vi "PPG_ABC.start ABC.vi"(0 "i ref in":refnum<vi>, 2 "patternGroup":i32, 3 "ms timeout [ms]":i32=10000, 5 "error in (no error)":errorcluster) -> (14 "i ref out":refnum<vi>, 17 "timed out":bool, 19 "error out":errorcluster)   [LabVIEW 2014, in "PPG_ABC.lvlib"]
doc: "Starts execution for the specified pattern group."
uses:
  PPG_ABC.lvlib
  PPG_ABC.PG_Running.ctl
  NI_FPGA_PPG/NI_FPGA_PPG.lvlib
  CSlibraries/UtilityLib/UtilityLib.lvlib
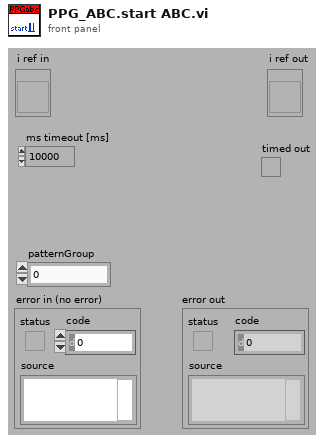
[diagram p1: front panel]
types:
  T1 = typedef "PPG_ABC.lvlib/PPG_ABC.PG_Running.ctl" = i32
  T2 = typedef "PPG_ABC.lvlib/PPG_ABC.i attribute.ctl" = cluster{"patternGroups":T3[], "defaultLetter":string, "defaultPatternGroup":i32, "PGRunning":T1, "PGRunningID":i32, "pgStarting":T4}
  T3 = typedef "PPG_ABC.lvlib/PPG_ABC.PG_dataType.ctl" = cluster{"PGDevice":string, "rawPatternData":cluster{"triggerCondition":i32, "timeTable":dbl[], "channelTable":string[]}[]}
  T4 = typedef "Semaphore RefNum" = refnum<k1>
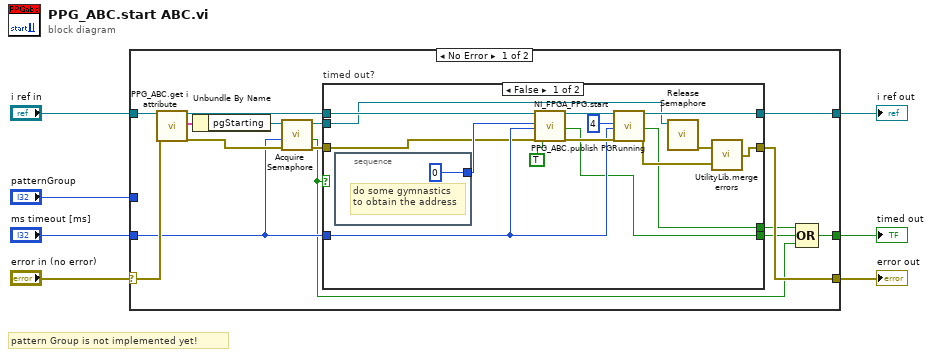
[diagram p0: block diagram]
diagram:
  # "pattern Group is not implemented yet!"
  n1 = case shown="No Error" "error in (no error)" {
    selector: "error in (no error)" -> [w19 w42]
    tunnel: [w21 w42] -> w6
    tunnel: "i ref in" -> [w20 w41]
    tunnel: [w22 w41] -> w4
    tunnel: [w10 _] -> w3
    tunnel: "ms timeout [ms]" -> [w12 _]
    tunnel: "patternGroup" -> [_ _]
    frame No Error {
      n2 = call "PPG_ABC.get i attribute.vi"("i ref in"=w20, "error in (no error)"=w19) -> ("i ref out"=w15:refnum<vi>, "i attribute"=w18:T2, "error out"=w16:errorcluster)  [unwired: 15 in]
      n3 = Unbundle By Name(w18) -> ("pgStarting"=w17:T4)
      n4 = call <vilib>:"Acquire Semaphore.vi"("error in (no error)"=w16, "ms timeout (-1)"=w12, "semaphore"=w17) -> ("error out"=w14:errorcluster, "timed out"=w11:bool, "semaphore out"=w13:T4)  [unwired: 2 in]
      n5 = case "timed out?" shown="False" w11 {
        tunnel: [w35 w40] -> w22
        tunnel: [w26 w39] -> w21
        tunnel: w12 -> [w33 _]
        tunnel: w15 -> [w31 w40]
        tunnel: w14 -> [w29 w39]
        tunnel: w13 -> [w30 _]
        tunnel: [w25 _] -> w9
        tunnel: [w24 _] -> w8
        frame False {
          n6 = stacked-sequence {
            tunnel: [0 ("start_addr")] -> w37
            frame #0 {
              # "do some gymnastics\nto obtain the address"
            }
          }
          n7 = call "NI_FPGA_PPG.start.vi"("i ref in"=w31, "start_addr"=w37, "ms timeout (10000)"=w33, "error in (no error)"=w29, "ignorePdcHandling"=TRUE) -> ("i ref out"=w36:refnum<vi>, "timed out"=w24:bool, "error out"=w34:errorcluster)  [unwired: 12 in]
          n8 = call "PPG_ABC.publish PGRunning.vi"("i ref in"=w36, "PPGRunning"=T1 4, "ms timeout (10000)"=w33, "error in (no error)"=w34) -> ("i ref out"=w35:refnum<vi>, "timed out"=w25:bool, "error out"=w27:errorcluster)  [unwired: 13 in]
          n9 = call <vilib>:"Release Semaphore.vi"("semaphore"=w30) -> ("error out"=w28:errorcluster)  [unwired: 5 in, 1 out]
          n10 = call "UtilityLib.merge errors.vi"("error2 (no error)"=w27, "error1 (no error)"=w28) -> ("error out"=w26:errorcluster)
        }
        frame True {
        }
      }
      n11 = Compound Arithmetic op=OR(w9, w8, w11) -> (w10:bool)
    }
    frame Error {
    }
  }
  "error out" <- w6
  "i ref out" <- w4
  "timed out" <- w3
